vi "DeltaMulti.vi"() -> ()   [LabVIEW 2019]
uses:
  Global 2.vi
panel:
  in  "Arm":bool
  in  "Measure":bool
  in  "Comp":dbl
  in  "Delay":dbl
  in  "I_Max":dbl
  out "T":cluster{"X":dbl[], "Y":dbl[]}[](graph)=[{"X"=[158.55365709999998, 159.610163, 160.67648119999998, 161.7360579, 162.7961535, 163.85780699999998], "Y"=[1.4652, 1.4652, 1.4653, 1.4652, 1.4651, 1.4652]}, {"X"=[158.55365709999998, 159.610163, 160.67648119999998, 161.7360579, 162.7961535, 163.85780699999998], "Y"=[1.6459, 1.6456, 1.6455, 1.6454, 1.6452, 1.6452]}] caption="XY Graph"
  in  "Reset":bool
  out "Sample Temp [K]":dbl
  out "Delta Reading [Ohm]":dbl=1.19099581
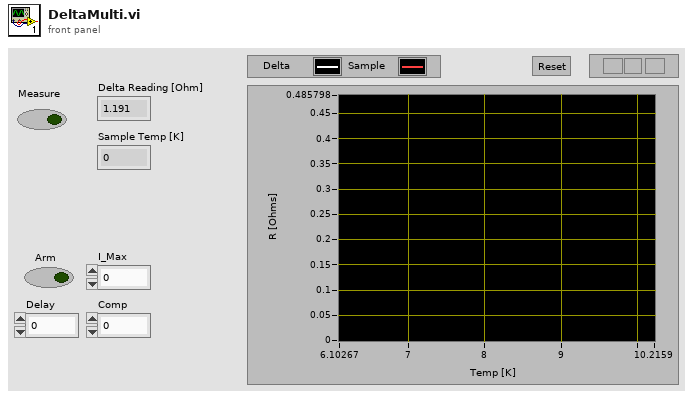
[diagram p1: front panel]
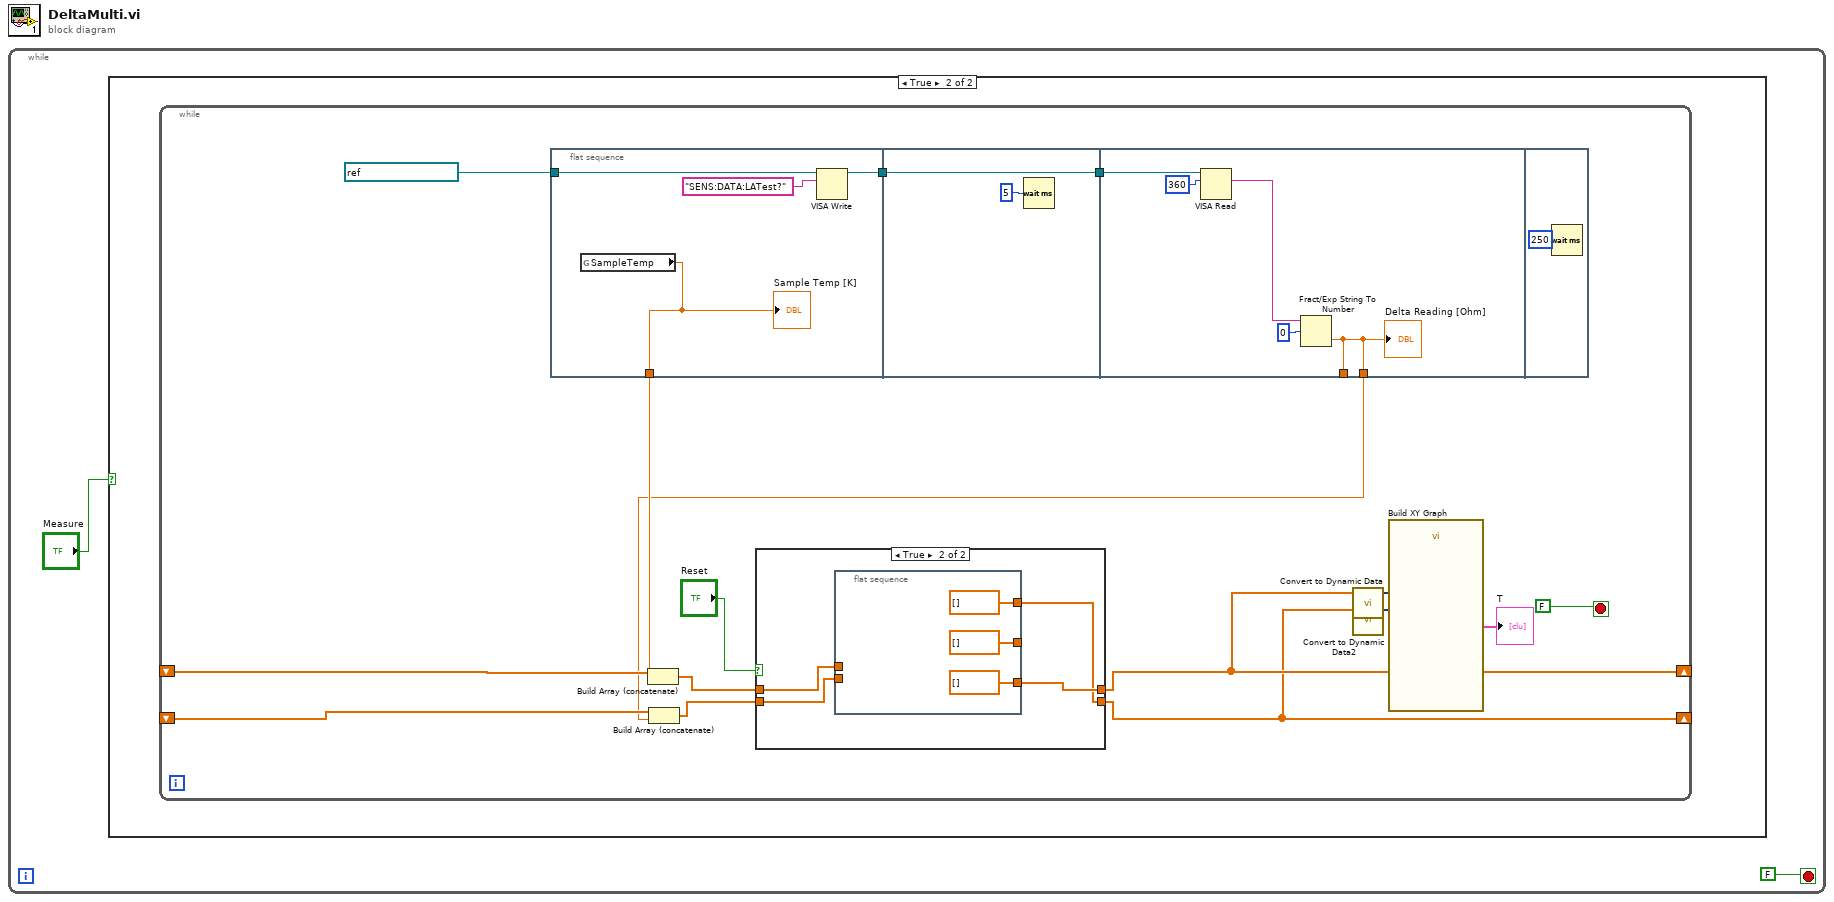
[diagram p0: block diagram]
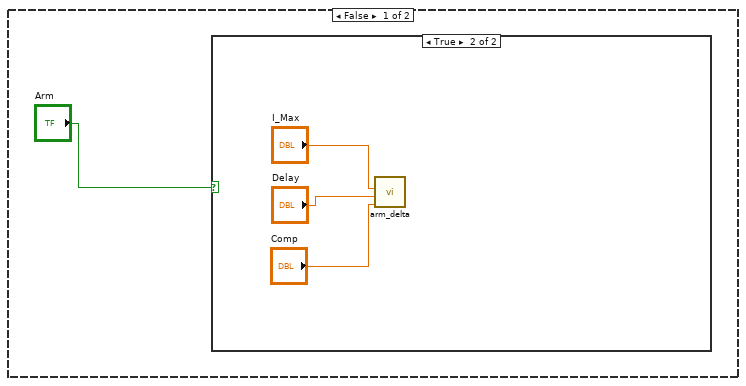
[diagram p2: hidden frame]
diagram:
  n1 = while {
    stop <- FALSE stop-if-true
    n2 = case shown="True" "Measure" {
      frame False {
        n3 = case shown="True" "Arm" {
          frame False {
          }
          frame True {
            n4 = call "arm_delta.vi"("Compliance [V]"="Comp", "DELAY [sec]"="Delay", "I-HIGH [A]"="I_Max") -> ()  [unwired: 9 in]
          }
        }
      }
      frame True {
        n5 = while {
          shift-right: [w10] -> _
          shift-left: _ -> [w18]
          shift-right: [w8] -> _
          shift-left: _ -> [w16]
          stop <- FALSE stop-if-true
          n6 = flat-sequence {
            tunnel: [w34] -> w22
            tunnel: refnum<visa-resource-name> "GPIB1::20::INSTR" ("Keithley") -> [w33]
            tunnel: [w32] -> w14
            tunnel: [w36] -> w21
            tunnel: w22 -> [w36]
            tunnel: [w38] -> _
            tunnel: w21 -> [w39]
            tunnel: [w38] -> w13
            frame #0 {
              n7 = global read "Global 2.vi" "SampleTemp"() -> (w32:dbl)
              "Sample Temp [K]" <- w32
              n8 = VISA Write(VISA resource name=w33, write buffer="SENS:DATA:LATest?" ("write buffer 2")) -> (VISA resource name out=w34:refnum<visa-resource-name>)  [unwired: 1 in, 2 out]
            }
            frame #1 {
              n9 = Wait (ms)(milliseconds to wait=5) -> ()  [unwired: 1 out]
            }
            frame #2 {
              n10 = VISA Read(VISA resource name=w39, byte count=u32 360) -> (read buffer=w41:string)  [unwired: 1 in, 3 out]
              n11 = Fract/Exp String To Number(string=w41, offset=0) -> (number=w38:dbl)  [unwired: 3 out]
              "Delta Reading [Ohm]" <- w38
            }
            frame #3 {
              n12 = Wait (ms)(milliseconds to wait=250) -> ()  [unwired: 1 out]
            }
          }
          n13 = Build Array (concatenate)(w18, w14) -> (w17:dbl[])
          n14 = Build Array (concatenate)(w16, w13) -> (w15:dbl[])
          n15 = case shown="True" "Reset" {
            tunnel: w17 -> [w24 w28]
            tunnel: [w24 w27] -> w10
            tunnel: w15 -> [w23 w26]
            tunnel: [w23 w25] -> w8
            frame False {
            }
            frame True {
              n16 = flat-sequence {
                tunnel: w28 -> [_]
                tunnel: w26 -> [_]
                tunnel: [dbl[] []] -> w25
                tunnel: [dbl[] []] -> w27
                tunnel: [dbl[] []] -> _
                frame #0 {
                }
              }
            }
          }
          n17 = call "Convert to Dynamic Data"("Array"=w10) -> ("Dynamic Data Type"=w9:dynamicdata)  [unwired: 3 in]
          n18 = call "Convert to Dynamic Data2"("Array"=w8) -> ("Dynamic Data Type"=w7:dynamicdata)  [unwired: 3 in]
          n19 = call "Build XY Graph"("Y Input"=w7, "X Input"=w9) -> ("XY Graph"=→"T":cluster{"X":dbl[], "Y":dbl[]}[])  [unwired: 8 in, 1 out]
        }
      }
    }
  }
